vi "Output on.vi"(8 "error in (no error)":errorcluster, 10 "Output On":bool, 11 "Agilent 6xxx in":refnum<class "Agilent 6xxx.lvclass">) -> (0 "error out":errorcluster, 3 "Agilent 6xxx out":refnum<class "Agilent 6xxx.lvclass">)   [LabVIEW 2020, in "Agilent 6xxx.lvclass"]
uses:
  Agilent 6xxx.lvclass
  C:/Sandbox/RF Bench/Source Code/WiSpry Test Framework/Instruments/Instrument.lvclass
  C:/Sandbox/RF Bench/Source Code/WiSpry Test Framework/Instruments/Power Supply/Power Supply.lvclass
  Power Supply.lvclass/Power Supply.ctl
  Instrument.lvclass/Instrument.ctl
  <instrlib>/Agilent 6XXX Series/Agilent 6XXX Series.lvlib
  Power Supply.lvclass
  Instrument.lvclass
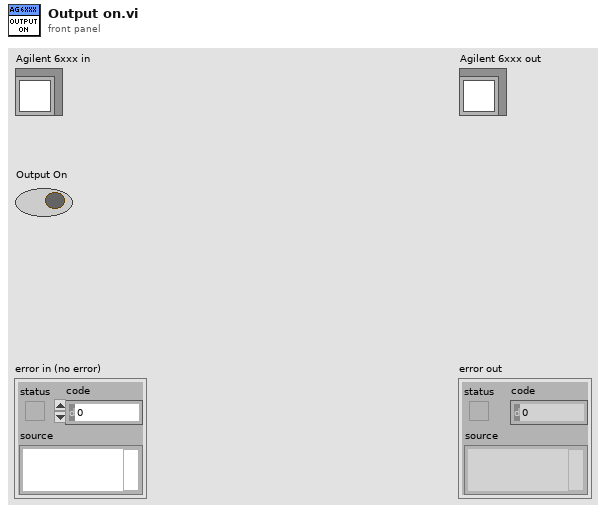
[diagram p1: front panel]
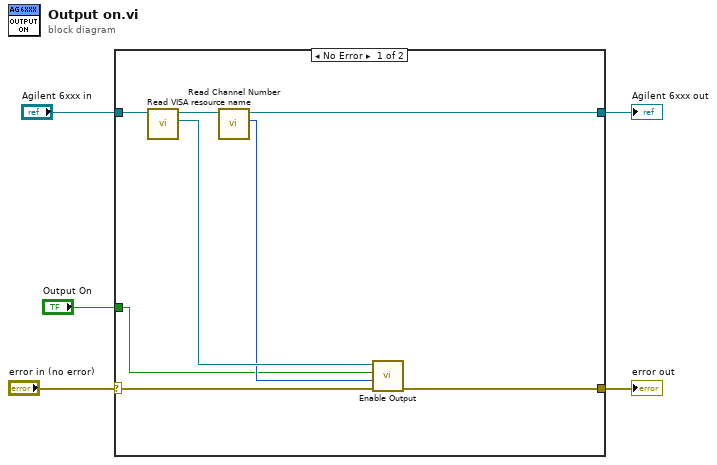
[diagram p0: block diagram]
diagram:
  n1 = case shown="No Error" "error in (no error)" {
    selector: "error in (no error)" -> [w7 w14]
    tunnel: [w11 w15] -> w5
    tunnel: "Agilent 6xxx in" -> [w12 w15]
    tunnel: [w6 w14] -> w2
    tunnel: "Output On" -> [w8 _]
    frame No Error {
      n2 = call "Read VISA resource name.vi"("Instrument in"=w12) -> ("VISA resource name"=w10:refnum<visa-resource-name>, "Instrument out"=w13:refnum<class "Agilent 6xxx.lvclass">)  [unwired: 9 in]
      n3 = call "Read Channel Number.vi"("Power Supply in"=w13) -> ("Channel Number"=w9:u8, "Power Supply out"=w11:refnum<class "Agilent 6xxx.lvclass">)  [unwired: 9 in]
      n4 = call <instrlib>:"Enable Output.vi"("error in (no error)"=w7, "channel (1)"=w9, "output (T:on)"=w8, "VISA resource name"=w10) -> ("error out"=w6:errorcluster)  [unwired: 6 in, 1 out]
    }
    frame Error {
    }
  }
  "error out" <- w2
  "Agilent 6xxx out" <- w5
